vi "OmniBus Example 1.vi"() -> ()   [LabVIEW 2021]
doc: "Omni-Bus 2.0.1.6\nTim - TSA\nCopyright (c) 2024, TSA"
uses:
  <vilib>/TSA/Omni-Bus/Omni-Bus/Omni_Bus.lvclass
  <vilib>/TSA/Omni-Bus/Omni-Bus/Support/Broad Types.ctl
  FPGA-Bus.lvclass
  C:/Program Files (x86)/National Instruments/LabVIEW 2021/vi.lib/TSA/Omni-Bus/Omni-Bus/Bus Access/Bus_Access.lvclass
  <vilib>/TSA/Omni-Bus/Omni-Bus/Support/Write As/Write SGL as Numeric.vi
  <vilib>/TSA/Omni-Bus/Omni-Bus/Support/Read As/Read Numeric as SGL.vi
  <vilib>/TSA/Abstract Data Classes/Abs_Types/Numeric/Abs_Numeric.lvclass
  C:/Program Files (x86)/National Instruments/LabVIEW 2021/vi.lib/TSA/Abstract Data Classes/Abs_Types/Type/Abs_Type.lvclass
  <vilib>/FPGAPlugInAG/cRIO-9053/niLvFpga_Open_cRIO-9053.vi
  <vilib>/rvi/interface/common/dynamic/niFpgaDynamicAddResources.vi
  <vilib>/TSA/Omni-Bus/Omni-Bus/Support/FindVar.vi
  <vilib>/rvi/interface/nirviOpenFPGA/nirviOpenFPGA.xnode
  FPGA Bitfiles/fpga-bus_FPGATarget_ExampleFPGAMain.lvbitx
panel:
  out "Read error":errorcluster
  out "Write error":errorcluster
  in  "Write Numeric":sgl
  in  "Write Tag":string(combo)
  in  "stop":bool
  out "Read Numeric":sgl format="%.2p"
  in  "Read Tag":string(combo)
  out "error out":errorcluster
  out "All Tags":string[](array[string])
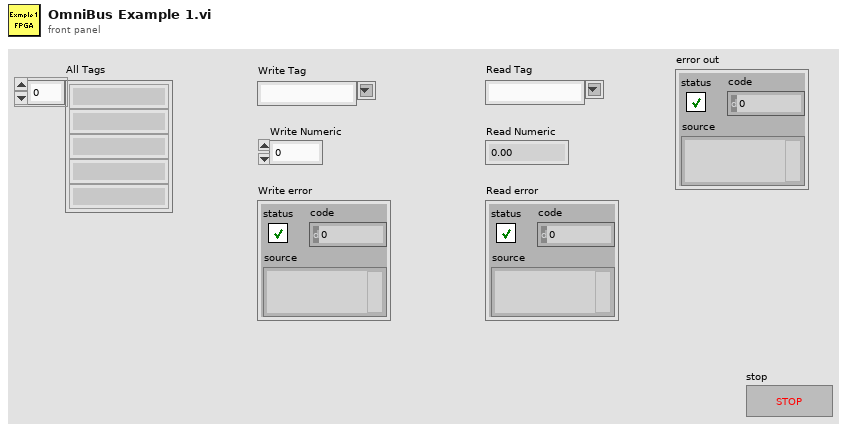
[diagram p1: front panel]
types:
  T1 = typedef "Omni_Bus.lvclass/Broad Types.ctl" = enum16{"All Tags", "NI Specific Type", "Boolean", "String", "Numeric", "Float", "Integer", "Collection", "All Value Types", "Non Value Types"}
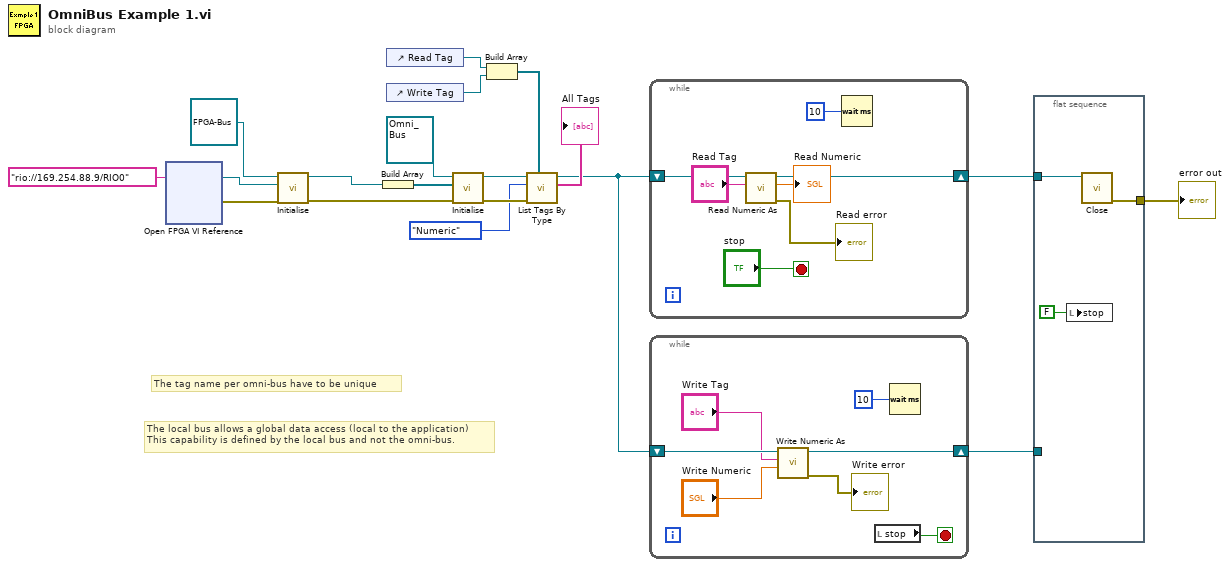
[diagram p0: block diagram]
diagram:
  # "The local bus allows a global data access (local to the application)\nThis capability is defined by the local bus and not the omni-bus."
  # "The tag name per omni-bus have to be unique"
  n1 = xnode "Open FPGA VI Reference"("resource name"=tag "rio://169.254.88.9/RIO0") -> ("FPGA VI Reference Out"=w3:refnum<k20>, "error out"=w1:errorcluster)  [unwired: 1 in]
  n2 = call "Initialise.vi"("error in (no error)"=w1, "FPGA Interface"=w3, "FPGA-Bus in"=refnum<class "FPGA-Bus.lvclass"> refnum ("FPGA-Bus.lvclass")) -> ("error out"=w9:errorcluster, "FPGA-Bus out"=w8:refnum<class "FPGA-Bus.lvclass">)  [unwired: 7 in]
  n3 = Build Array(w8) -> (w18:refnum<class "FPGA-Bus.lvclass">[])
  n4 = control-ref of="Read Tag"() -> (w6:refnum<vi>)
  n5 = control-ref of="Write Tag"() -> (w5:refnum<vi>)
  n6 = call-dynamic "Initialise.vi"("error in (no error)"=w9, "Bus Access"=w18, "Var Bus in"=refnum<class "Omni_Bus.lvclass"> refnum) -> ("error out"=w16:errorcluster, "Var Bus out"=w17:refnum<class "Omni_Bus.lvclass">)  [unwired: 7 in]
  n7 = Build Array(w6, w5) -> (w4:refnum<vi>[])
  n8 = call <vilib>:"List Tags By Type.vi"("Combo Boxes"=w4, "error in (no error)"=w16, "Broad Types"=Broad_Types."Numeric", "Var Bus in"=w17) -> ("Tags"=→"All Tags":string[], "Var Bus out"=w11:refnum<class "Omni_Bus.lvclass">)  [unwired: 4 in, 2 out]
  n9 = while {
    shift-right: [w25] -> w12
    shift-left: w11 -> [w26]
    stop <- "stop" stop-if-true
    n10 = call-poly <vilib>:"Read Numeric As.vi"("Tag"="Read Tag", "Var Bus in"=w26) -> ("error out"=→"Read error":errorcluster, "Numeric"=→"Read Numeric":sgl, "Var Bus out"=w25:refnum<class "Omni_Bus.lvclass">)  [unwired: 7 in]
    n11 = Wait (ms)(milliseconds to wait=u32 10) -> ()  [unwired: 1 out]
  }
  n12 = while {
    shift-right: [w32] -> w10
    shift-left: w11 -> [w33]
    stop <- w29 stop-if-true
    n13 = call-poly <vilib>:"Write Numeric As.vi"("Numeric"="Write Numeric", "Tag"="Write Tag", "Omni_Bus in"=w33) -> ("error out"=→"Write error":errorcluster, "Omni_Bus out"=w32:refnum<class "Omni_Bus.lvclass">)  [unwired: 7 in]
    n14 = local read "stop"() -> (w29:bool)
    n15 = Wait (ms)(milliseconds to wait=u32 10) -> ()  [unwired: 1 out]
  }
  n16 = flat-sequence {
    tunnel: [w36] -> w13
    tunnel: w12 -> [w35]
    tunnel: w10 -> [_]
    frame #0 {
      n17 = local write "stop"(FALSE ("stop")) -> ()
      n18 = call-dynamic "Close.vi"("Data in"=w35) -> ("error out"=w36:errorcluster)  [unwired: 9 in, 1 out]
    }
  }
  "error out" <- w13
